vi "Discover roboRIO.vi"(8 "error in (no error)":errorcluster) -> (0 "error out":errorcluster, 2 "roboRIO IP address":string, 3 "roboRIO name":string)   [LabVIEW 2018]
doc: "Use this VI to discover a roboRIO connected to the computer."
uses:
  <vilib>/nisyscfg/Close (System).vi
  <vilib>/nisyscfg/nisyscfg.lvlib
  <resource>/objmgr/nisysapi.rc
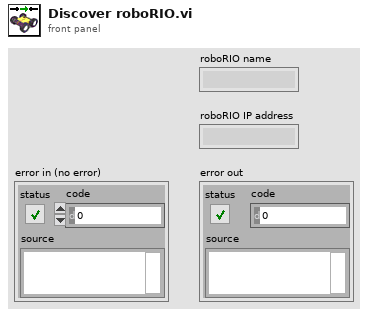
[diagram p1: front panel]
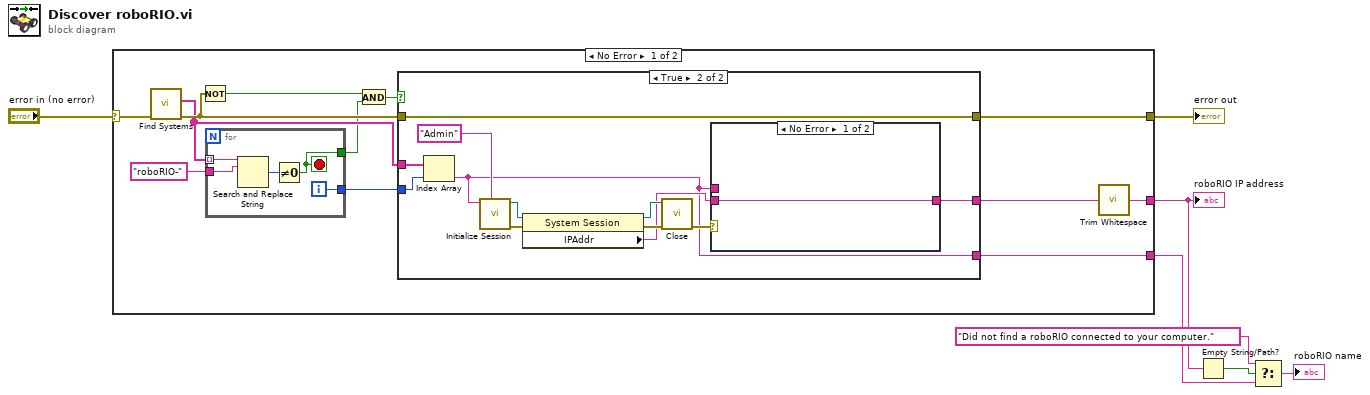
[diagram p0: block diagram]
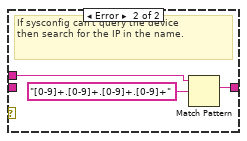
[diagram p3: hidden frame]
diagram:
  n1 = case shown="No Error" "error in (no error)" {
    selector: "error in (no error)" -> [w15 w42]
    tunnel: [w19 w42] -> w7
    tunnel: [w8 _] -> w5
    tunnel: [w16 _] -> w2
    frame No Error {
      n2 = call <vilib>:"Find Systems.vi"("error in (no error)"=w15) -> ("error out"=w18:errorcluster, "Detected Systems"=w13:string[])  [unwired: 8 in, 1 out]
      n3 = Not(x=w18) -> (.not. x?=w9:bool)
      n4 = for {
        tunnel: w13 -> [w41] mode=indexing
        tunnel: "roboRIO-" ("string") -> [w40]
        tunnel: [w38] -> w12
        tunnel: [w37] -> w11
        i -> [w37]
        stop <- w38 stop-if-true
        n5 = Search and Replace String(input string=w41, search string=w40) -> (number of replacements=w39:i32)  [unwired: 6 in, 3 out]
        n6 = Not Equal To 0?(x=w39) -> (x != 0?=w38:bool)
      }
      n7 = And(x=w9, y=w12) -> (x .and. y?=w10:bool)
      n8 = case shown="True" w10 {
        tunnel: w13 -> [_ w27]
        tunnel: w11 -> [_ w26]
        tunnel: [_ w22] -> w16
        tunnel: [_ w24] -> w17
        tunnel: w18 -> [w20 w21]
        tunnel: [w20 w21] -> w19
        frame False {
        }
        frame True {
          n9 = Index Array(array=w27, index=w26) -> (element=w22:string)
          n10 = call <vilib>:"Initialize Session.vi"("User Name"="Admin", "Target (localhost)"=w22) -> ("error out"=w31:errorcluster, "Session out"=w32:refnum<k21>)  [unwired: 8 in]
          n11 = property class="System Session"(reference=w32, error in=w31) -> (reference out=w30:refnum<k21>, error out=w29:errorcluster, "IPAddr"=w23:string)
          n12 = call-poly <vilib>:"Close.vi"("error in (no error)"=w29, "Session in"=w30) -> ("error out"=w25:errorcluster)  [unwired: 9 in]
          n13 = case shown="No Error" w25 {
            tunnel: [w33 w34] -> w24
            tunnel: w23 -> [w33 _]
            tunnel: w22 -> [_ w36]
            frame No Error {
            }
            frame Error {
              # "If sysconfig can't query the device\nthen search for the IP in the name."
              n14 = Match Pattern(string=w36, regular expression="[0-9]+.[0-9]+.[0-9]+.[0-9]+") -> (match substring=w34:string)  [unwired: 1 in, 3 out]
            }
          }
        }
      }
      n15 = call <vilib>:"Trim Whitespace.vi"("string"=w17) -> ("trimmed string"=w8:string)  [unwired: 1 in]
    }
    frame Error {
    }
  }
  "error out" <- w7
  "roboRIO IP address" <- w5
  n16 = Empty String/Path?(string/path=w5) -> (empty?=w4:bool)
  n17 = Select(t="Did not find a roboRIO connected to your computer.", s=w4, f=w2) -> (s? t:f=→"roboRIO name":string)
